vi "Autonomous Independent.vi"() -> ()   [LabVIEW 2013]
doc: "This VI is called when autonomous begins, and will automatically be terminated when autonomous ends. You can carry out timed or sensor driven robot movement independently without needing to return to the caller."
uses:
  Robot Global Data.vi
panel:
  in  "Please Put Here Camera Sonar Value Global 2":dbl
  in  "Please Put Here Camera Sonar Value Global":dbl
  in  "Distance wanted (ft)":dbl=6.0 format="%#_13g"
  # "Be sure to right-click and choose Data Operations>>Make Current Value default if you want to save the array values with the VI"
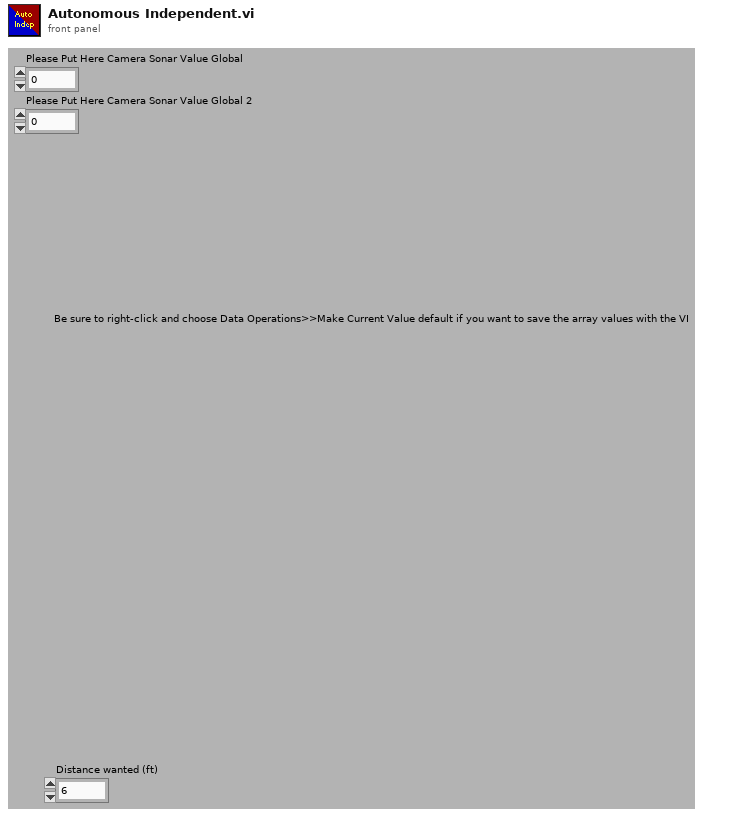
[diagram p1: front panel]
types:
  T1 = typedef "WPI_ServoDeviceRef.ctl" = cluster{"DeviceStatus":errorcluster, "Digital Module":T2, "PWM Channel":T3, "DeadBand":T4}
  T2 = typedef "FPGA_TypedefDigitalModule.ctl" = enum16{"Digital Module 1", "Digital Module 2"}
  T3 = typedef "FPGA_DIOPWMChannel.ctl" = enum8{"PWM 1", "PWM 2", "PWM 3", "PWM 4", "PWM 5", "PWM 6", "PWM 7", "PWM 8", "PWM 9", "PWM 10", "Invalid"}
  T4 = typedef "WPI_PWMDeadband.ctl" = cluster{"Name":string, "maxPositivePwm":i32, "minPositivePwm":i32, "centerPwm":i32, "maxNegativePwm":i32, "minNegativePwm":i32, "angularRange":u16}
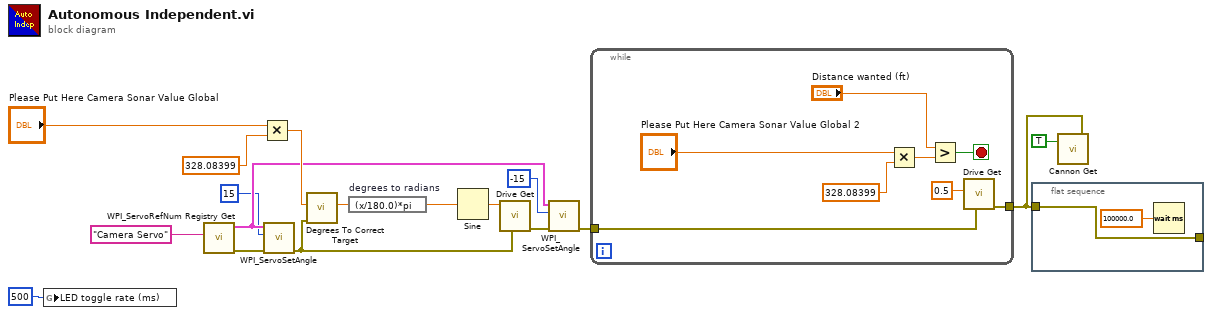
[diagram p0: block diagram]
diagram:
  n1 = global write "Robot Global Data.vi" "LED toggle rate (ms)"(u32 500 ("LED ms toggle rate")) -> ()
  n2 = call <vilib>:"WPI_ServoRefNum Registry Get.vi"("refnum name"="Camera Servo") -> ("error out"=w8:errorcluster, "ServoDeviceRef"=w12:T1)  [unwired: 9 in]
  n3 = Multiply(x="Please Put Here Camera Sonar Value Global", y=328.08399) -> (x*y=w13:dbl)
  n4 = call <vilib>:"WPI_ServoSetAngle.vi"("error in (no error)"=w8, "Angle"=15, "ServoDeviceRef"=w12) -> ("error out"=w5:errorcluster)  [unwired: 7 in, 1 out]
  n5 = call "Degrees To Correct Target.vi"("error in"=w5, "Distance to Wall (ft)"=w13) -> ("Degrees"=w15:dbl)  [unwired: 8 in, 1 out]
  n6 = expression code="(x/180.0)*pi" "degrees to radians"(w15) -> (w16:dbl)
  n7 = Sine(x=w16) -> (sin(x)=w6:dbl)
  n8 = call "Drive Get.vi"("error in (no error)"=w5, "X - Axis"=w6) -> ("error out"=w4:errorcluster)  [unwired: 9 in]
  n9 = call <vilib>:"WPI_ServoSetAngle.vi"("error in (no error)"=w4, "Angle"=-15, "ServoDeviceRef"=w12) -> ("error out"=w7:errorcluster)  [unwired: 7 in, 1 out]
  n10 = while {
    tunnel: w7 -> [w20]
    tunnel: [w19] -> w1
    stop <- w24 stop-if-true
    n11 = Multiply(x="Please Put Here Camera Sonar Value Global 2", y=328.08399) -> (x*y=w22:dbl)
    n12 = Greater?(x="Distance wanted (ft)", y=w22) -> (0:w24:bool)
    n13 = call "Drive Get.vi"("error in (no error)"=w20, "Y - Axis"=0.5 ("Y axis value")) -> ("error out"=w19:errorcluster)  [unwired: 9 in]
  }
  n14 = flat-sequence {
    tunnel: w1 -> [w26]
    tunnel: [w26] -> _
    frame #0 {
      n15 = Wait (ms)(milliseconds to wait=100000.0) -> ()  [unwired: 1 out]
    }
  }
  n16 = call "Cannon Get.vi"("error in (no error)"=w1, "Le Fire At Will?"=TRUE) -> ()  [unwired: 1 in]
